vi "Register Generic gRPC Method.vi"(8 "error in (no error)":errorcluster, 11 "Template Server in":refnum<class "Template Server.lvclass">) -> (0 "error out":errorcluster, 3 "Template Server out":refnum<class "Template Server.lvclass">)   [LabVIEW 2019, in "Template Server.lvlib" / "Template Server.lvclass"]
uses:
  Template Server.lvclass
  gRPC lvSupport/gprc-lvsupport.lvlib
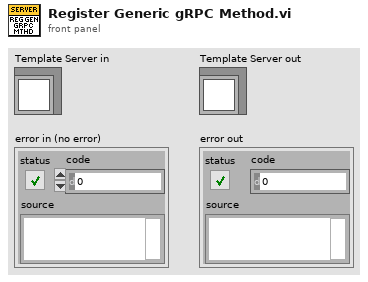
[diagram p1: front panel]
types:
  T1 = typedef "Template Server.lvlib/gprc-lvsupport.lvlib/grpcId.ctl" = u64
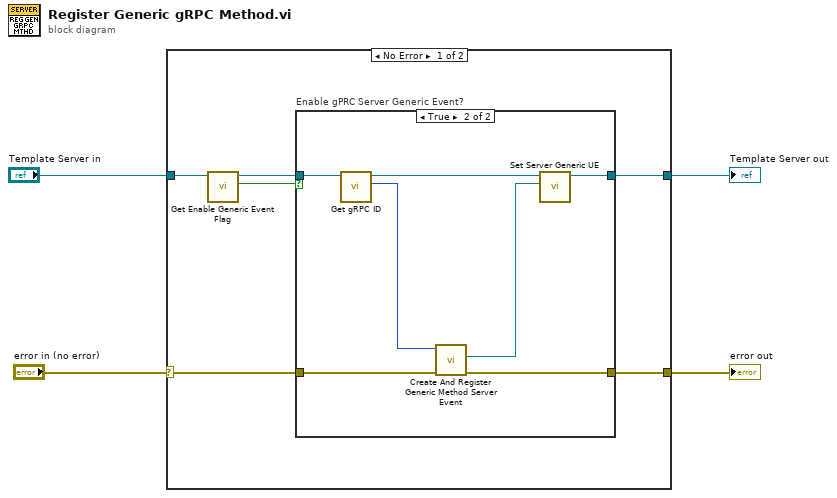
[diagram p0: block diagram]
diagram:
  n1 = case shown="No Error" "error in (no error)" {
    selector: "error in (no error)" -> [w10 w20]
    tunnel: "Template Server in" -> [w7 w21]
    tunnel: [w9 w20] -> w3
    tunnel: [w8 w21] -> w2
    frame No Error {
      n2 = call "Get Enable Generic Event Flag.vi"("Template Server in"=w7) -> ("Enable Generic Event Flag"=w5:bool, "Template Server out"=w6:refnum<class "Template Server.lvclass">)  [unwired: 9 in]
      n3 = case "Enable gPRC Server Generic Event?" shown="True" w5 {
        tunnel: w10 -> [w11 w19]
        tunnel: [w11 w18] -> w9
        tunnel: [w12 w15] -> w8
        tunnel: w6 -> [w12 w13]
        frame False {
        }
        frame True {
          n4 = call "Get gRPC ID.vi"("OOP Server in"=w13) -> ("gRPC ID"=w17:T1, "OOP Server out"=w16:refnum<class "Template Server.lvclass">)  [unwired: 9 in]
          n5 = call "Create And Register Generic Method Server Event.vi"("error in (no error)"=w19, "gRPCid server in"=w17) -> ("error out"=w18:errorcluster, "Generic Method Event"=w14:refnum<user-event>)  [unwired: 7 in, 1 out]
          n6 = call "Set Server Generic UE.vi"("Server Generic UE"=w14, "Template Server in"=w16) -> ("Template Server out"=w15:refnum<class "Template Server.lvclass">)  [unwired: 9 in]
        }
      }
    }
    frame Error {
    }
  }
  "error out" <- w3
  "Template Server out" <- w2
